vi "IMAQdx Wait for Frame Done.vi"(7 "Timeout (ms)":i32=5000, 8 "error in":errorcluster, 11 "Session In":T1) -> (0 "error out":errorcluster, 2 "Buffer Number":u32, 3 "Session Out":T1)   [LabVIEW 2020, in "NI_Vision_Acquisition_Software.lvlib"]
doc: "Synchronous wait for the next Frame Done event."
uses:
  NI_Vision_Acquisition_Software.lvlib
  IMAQdx.ctl
  niimaqdx.dll
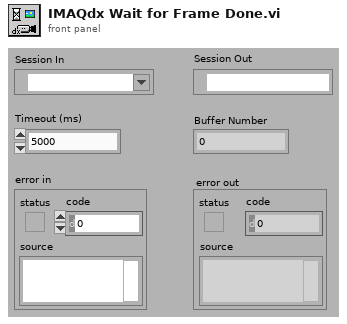
[diagram p1: front panel]
types:
  T1 = typedef "IMAQdx.ctl" = refnum<k21>
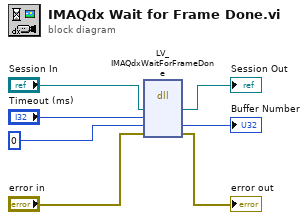
[diagram p0: block diagram]
diagram:
  n1 = dll-call lib="niimaqdx.dll" fn="LV_IMAQdxWaitForFrameDone"("refnum"="Session In", "timeoutMs"="Timeout (ms)", "bufferNumber"=u32 0, "error"="error in") -> ("refnum"=→"Session Out":T1, "bufferNumber"=→"Buffer Number":u32, "error"=→"error out":errorcluster)  [unwired: 5 in, 2 out]
